vi "Execute.vi"(8 "error in":errorcluster, 11 "STEP in":refnum<class "STEP.lvclass">) -> (0 "error out":errorcluster, 1 "Next Step?":bool, 2 "MSG":string, 3 "STEP out":refnum<class "STEP.lvclass">)   [LabVIEW 2015, in "Sequence Composition.lvlib" / "STEP.lvclass"]
uses:
  STEP.lvclass
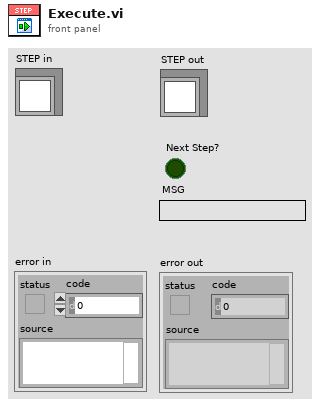
[diagram p1: front panel]
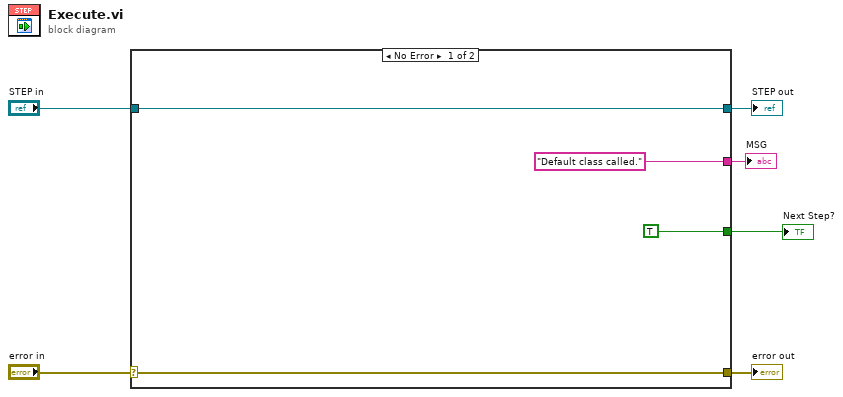
[diagram p0: block diagram]
diagram:
  n1 = case shown="No Error" "error in" {
    selector: "error in" -> [w9 w12]
    tunnel: [w9 w12] -> w5
    tunnel: [w10 w11] -> w3
    tunnel: "STEP in" -> [w10 w11]
    tunnel: [TRUE ("Next Step?") _] -> w2
    tunnel: ["Default class called." ("MSG") _] -> w1
    frame No Error {
    }
    frame Error {
    }
  }
  "error out" <- w5
  "STEP out" <- w3
  "Next Step?" <- w2
  "MSG" <- w1
